vi "Maxi Gauge - Example 2.vi"(8 "error in (no error)":errorcluster caption="Fehler (Eingang, kein Fehler)", 11 "input refnum":refnum<visa-resource-name> caption="Eingang (Referenz)") -> (0 "error out":errorcluster, 1 "Get Sensor Identification":T1, 2 "Get Channel Identification":T2)   [LabVIEW 2013, in "Maxi Gauge.lvlib"]
uses:
  <instrlib>/Maxi Gauge/Maxi Gauge.lvlib
panel:
  out "Unit Get":i8(ring)=1 items=["mbar", "Torr", "Pascal", "", ""]
  out "Digits Get":i8(ring)=1 items=["", "", "2", "3", ""]
  out "Baragraph Get":i8(ring)=1 items=["off", "Sensor-Range", "1 Decade", ""]
  in  "Unit Set":i8(ring)=4 items=["mbar", "Torr", "Pascal", "", ""]
  in  "Digits Set":i8(ring)=4 items=["", "", "2", "3", ""]
  in  "Baragraph Set":i8(ring)=3 items=["off", "Sensor-Range", "1 Decade", ""]
  in  "W/R 4":bool
  out "OFF Threshold Get:":dbl=1e-13 min=1e-13 max=41000.0 format="%.2e"
  out "ON Threshold Get:":dbl=1e-13 min=1e-13 max=41000.0 format="%.2e"
  out "Control Sensor OFF Get:":u8(ring) items=["sensor 1", "sensor 2", "sensor 3", "sensor 4", "sensor 5", "sensor 6", "Extern", "Manual", "Hotstart"]
  out "Control Sensor ON Get:":u8(ring) items=["sensor 1", "sensor 2", "sensor 3", "sensor 4", "sensor 5", "sensor 6", "Extern", "Manual", "Hotstart"]
  in  "Set Calibration factor":dbl=1.0 min=0.1 max=9.999 step=0.001 format="%.3f"
  in  "Set Contrast":i8=-1 min=-1 max=20 step=1
  in  "W/R 2":bool
  in  "Sensor Nr.:":i32(ring) items=["sensor 1", "sensor 2", "sensor 3", "sensor 4", "sensor 5", "sensor 6"]
  out "Get Calibration factor":dbl=0.000753 format="%.3f"
  out "Get Screensave":i8=-1 min=-1 max=99 step=1
  out "Get Contrast":i8=-1 min=-1 max=20 step=1
  in  "W/R":bool
  # "1"
  # "2"
  # "5"
  # "4"
  # "3"
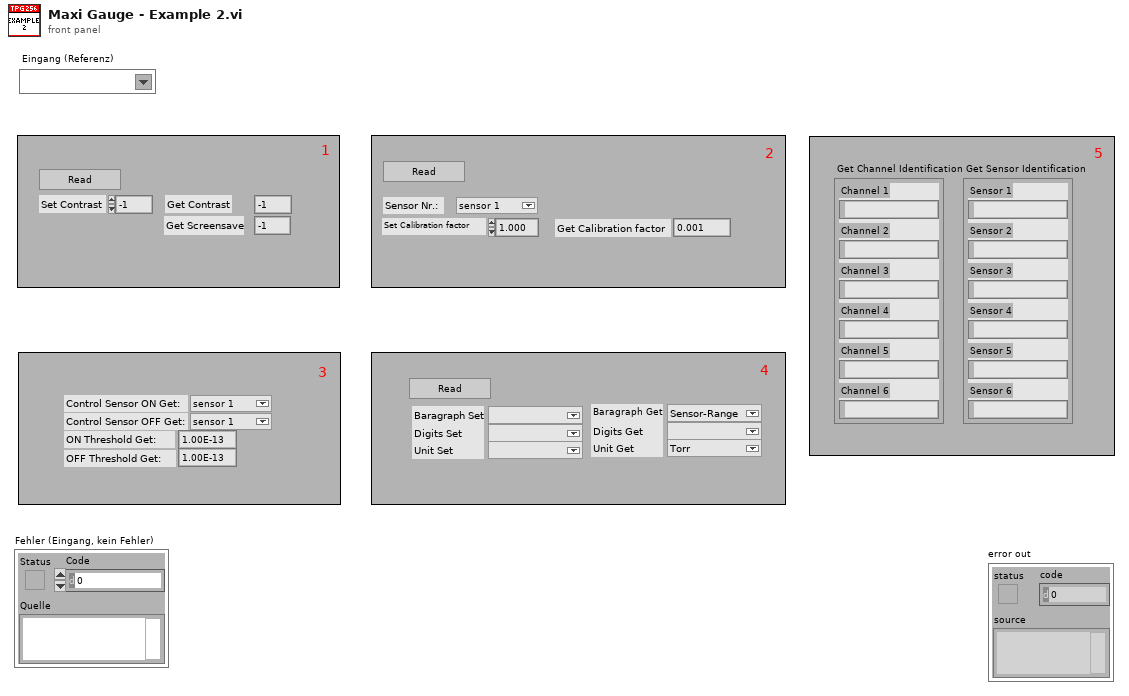
[diagram p1: front panel]
types:
  T1 = cluster{"Sensor 1":string, "Sensor 2":string, "Sensor 3":string, "Sensor 4":string, "Sensor 5":string, "Sensor 6":string}
  T2 = cluster{"Channel 1":string, "Channel 2":string, "Channel 3":string, "Channel 4":string, "Channel 5":string, "Channel 6":string}
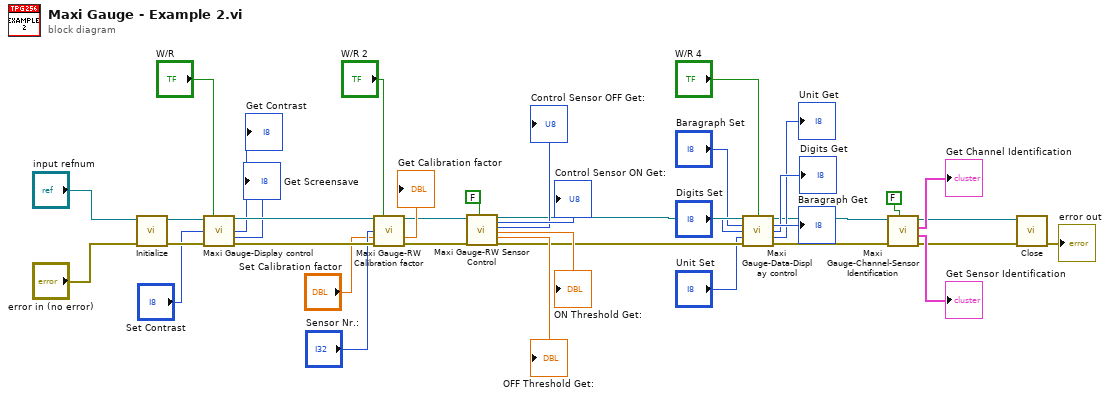
[diagram p0: block diagram]
diagram:
  n1 = call <instrlib>:"Initialize.vi"("error in (no error)"="error in (no error)", "input refnum"="input refnum") -> ("error out"=w37:errorcluster, "VISA resource out"=w38:refnum<visa-resource-name>)  [unwired: 8 in]
  n2 = call <instrlib>:"Maxi Gauge-Display control.vi"("VISA-Ressource in"=w38, "W/R"="W/R", "Set Contrast"="Set Contrast", "Fehler (Eingang)"=w37) -> ("VISA-Ressource out"=w35:refnum<visa-resource-name>, "Get Contrast"=→"Get Contrast":i8, "Get Screensave"=→"Get Screensave":i8, "Fehler (Ausgang)"=w36:errorcluster)  [unwired: 8 in]
  n3 = call <instrlib>:"Maxi Gauge-RW Calibration factor.vi"("VISA-Ressource in"=w35, "W/R"="W/R 2", "Sensor Nr.:"="Sensor Nr.:", "Set Calibration factor"="Set Calibration factor", "Fehler (Eingang)"=w36) -> ("VISA-Ressource out"=w24:refnum<visa-resource-name>, "Get Calibration factor"=→"Get Calibration factor":dbl, "Fehler (Ausgang)"=w23:errorcluster)  [unwired: 8 in]
  n4 = call <instrlib>:"Maxi Gauge-RW Sensor Control.vi"("VISA-Ressource in"=w24, "Fehler (Eingang, kein Fehler)"=w23, "W/R"=FALSE ("W/R 3")) -> ("VISA-Ressource out"=w17:refnum<visa-resource-name>, "Control Sensor ON Get:"=→"Control Sensor ON Get:":u8, "Control Sensor OFF Get:"=→"Control Sensor OFF Get:":u8, "ON Threshold Get:"=→"ON Threshold Get:":dbl, "OFF Threshold Get:"=→"OFF Threshold Get:":dbl, "Fehler (Ausgang)"=w16:errorcluster)  [unwired: 11 in]
  n5 = call <instrlib>:"Maxi Gauge-Data-Display control.vi"("VISA-Ressource in"=w17, "W/R"="W/R 4", "Baragraph Set"="Baragraph Set", "Digits Set"="Digits Set", "Unit Set"="Unit Set", "Fehler (Eingang)"=w16) -> ("VISA-Ressource out"=w7:refnum<visa-resource-name>, "Baragraph Get"=→"Baragraph Get":i8, "Digits Get"=→"Digits Get":i8, "Unit Get"=→"Unit Get":i8, "Fehler (Ausgang)"=w6:errorcluster)  [unwired: 5 in]
  n6 = call <instrlib>:"Maxi Gauge-Channel-Sensor Identification.vi"("W/R"=FALSE ("W/R 3"), "Fehler (Eingang, kein Fehler)"=w6, "VISA-Ressource in"=w7) -> ("Fehler (Ausgang)"=w1:errorcluster, "Get Sensor Identification"=→"Get Sensor Identification":T1, "Get Channel Identification"=→"Get Channel Identification":T2, "VISA-Ressource out"=w2:refnum<visa-resource-name>)  [unwired: 5 in]
  n7 = call <instrlib>:"Close.vi"("error in (no error)"=w1, "VISA resource name"=w2) -> ("error out"=→"error out":errorcluster)  [unwired: 9 in]
